vi "Recordings.vi"(1 "Data In":dbl[][](array[numeric]), 2 "Action":T1) -> (0 "Data Out":dbl[][](array[numeric]))   [LabVIEW 2013]
uses:
  Action.ctl
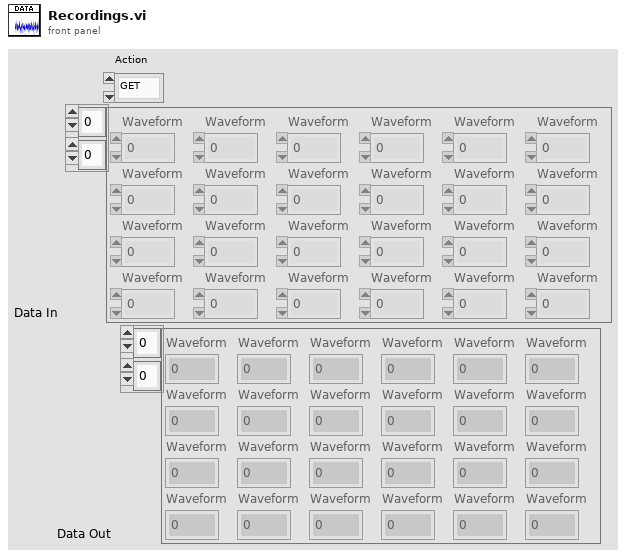
[diagram p1: front panel]
types:
  T1 = typedef "Action.ctl" = enum16{"GET", "PUT", "DELETE"}
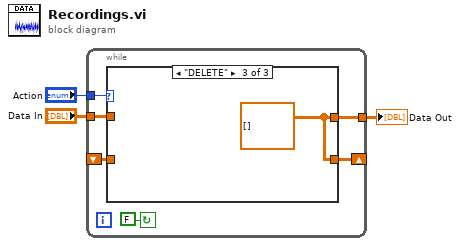
[diagram p0: block diagram]
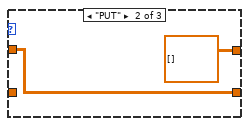
[diagram p3: hidden frame]
diagram:
  n1 = while {
    tunnel: "Action" -> [w8]
    tunnel: "Data In" -> [w7]
    shift-right: [w6] -> _
    shift-left: _ -> [w5]
    tunnel: [w4] -> w1
    stop <- FALSE continue-if-true
    n2 = case shown="\"DELETE\"" w8 {
      tunnel: w7 -> [_ w12 _]
      tunnel: [w10 w12 w13] -> w6
      tunnel: w5 -> [w10 _ _]
      tunnel: [w10 dbl[][] [] ("Data In") w13] -> w4
      frame "GET", Default {
      }
      frame "PUT" {
      }
      frame "DELETE" {
        w13 = dbl[][] [] ("Data In")
      }
    }
  }
  "Data Out" <- w1
